vi "radar.vi"(0 "Radar configuration":string="{\n\t\"type\": \"Radar\",\n\t\"gpu_number\": 0,\n\t\"listen_port\": 8302,\n\t\"send_radar_cube\": false,\n\t\"paint_targets\": false,\n\t\"run_tracker\": true,\n\t\"tracker\": {\n\t\t\"cluster_threshold\": 1.0,\n\t\t\"filter_size\": 8,\n\t\t\"kalman_alpha\": 10.0,\n\t\t\"kinematic_iir_alpha\": 0.05000000074505806,\n\t\t\"min_cluster_distance\": 25.0,\n\t\t\"min_detections_per_cluster\": 2,\n\t\t\"missed_detections_threshold\": 5,\n\t\t\"vel_coeff\": 0.699999988079071,\n\t\t\"write_debug_json\": \"\",\n\t\t\"x_dir_coeff\": 9.0,\n\t\t\"y_dir_coeff\": 4.199999809265137\n\t},\n\t\"rois\": [{\n\t\t\"max_angle\": 10.0,\n\t\t\"max_range\": 20.0,\n\t\t\"min_angle\": 0.0,\n\t\t\"min_range\": 1.0,\n\t\t\"roi_name\": \"test_left_roi\"\n\t}, {\n\t\t\"max_angle\": 0.0,\n\t\t\"max_range\": 20.0,\n\t\t\"min_angle\": -10.0,\n\t\t\"min_range\": 1.0,\n\t\t\"roi_name\": \"test_right_roi\"\n\t}],\n\t\"target_paint_lifetime\": 0.5,\n\t\"nearest_target_label_radius\": 100.0,\n\t\"location\": {\n\t\t\"x\": 245.0,\n\t\t\"y\": 0.0,\n\t\t\"z\": 40.0\n\t},\n\t\"rotation\": {\n\t\t\"pitch\": 0.0,\n\t\t\"yaw\": 0.0,\n\t\t\"roll\": 0.0\n\t},\n\t\"num_samples_per_sweep\": 345,\n\t\"fs\": 50000000,\n\t\"fc\": 77000000000.0,\n\t\"num_sweeps\": 16,\n\t\"sweep_time\": 0.0000069,\n\t\"bandwidth\": 250000000,\n\t\"max_radar_returns\": 500,\n\t\"elements\": 8,\n\t\"transmitter\": {\n\t\t\"peak_power\": 5.0,\n\t\t\"aperture\": 0.000859,\n\t\t\"gain\": 13.50\n\t},\n\t\"receiver\": {\n\t\t\"aperture\": 0.000798,\n\t\t\"nf\": 10.0,\n\t\t\"noise_temp\": 290.0,\n\t\t\"nb\": 74000000.0,\n\t\t\"gain\": 10.0\n\t},\n\t\"sbr\": {\n\t\t\"long_range_scan_distance\": 100.0,\n\t\t\"short_range_scan_distance\": 30.0,\n\t\t\"long_range_fov\": 30.0,\n\t\t\"short_range_fov\": 60.0,\n\t\t\"elevation_fov\": 10.0,\n\t\t\"ray_division_y\": 10.0,\n\t\t\"ray_division_z\": 10.0,\n\t\t\"debug_frustum\": false,\n\t\t\"debug_scan\": false,\n\t\t\"debug_rescan\": false\n\t}\n}", 3 "error in":errorcluster) -> (4 "Radar configuration":string="[\n    {\n  \"type\": \"Radar\",\n  \"packet_size\": 64000,\n   \"gpu_number\":0,\n  \"listen_port\": 8301,\n  \"synchronized_display\": true,\n  \"paint_targets\": false,\n  \"target_paint_lifetime\": 0.5,\n  \"location\": {\n    \"x\": 250.0,\n    \"y\": 0.0,\n    \"z\": 50.0\n  },\n  \"rotation\": {\n    \"pitch\": 0.0,\n    \"yaw\": 0.0,\n    \"roll\": 0.0\n  },\n  \"num_samples_per_sweep\":345,\n  \"fs\": 50000000,\n  \"fc\": 77000000000.0,\n  \"num_sweeps\": 32,\n  \"sweep_time\" : 0.0000069,\n  \"bandwidth\" : 172500000,\n  \"max_targets\": 250,\n  \"elements\": 8,\n  \"transmitter\": {\n    \"peak_power\": 5.0,\n    \"aperture\": 0.000859,\n    \"gain\": 13.50\n  },\n  \"receiver\": {\n    \"aperture\": 0.000798,\n    \"nf\": 10.0,\n    \"noise_temp\": 290.0,\n    \"nb\": 74000000.0,\n    \"gain\": 10.0\n  },\n  \"sbr\": {\n    \"long_range_scan_distance\": 150.0,\n    \"short_range_scan_distance\": 60.0,\n    \"long_range_fov\": 20.0,\n    \"short_range_fov\": 60.0,\n    \"elevation_fov\": 10.0,\n    \"rescan_density\": 20.0,\n    \"debug_frustum\": false,\n    \"debug_scan\": false,\n    \"debug_rescan\": false\n  }\n}\n]", 5 "Radar Sample":T2, 6 "Radar Data Cube":string, 7 "Target list":string, 8 "error out":errorcluster)   [LabVIEW 2019]
doc: "Configure and reads the data stream for the Radar sensor.\ns"
uses:
  tools/simx_common.vi
  controls/radarSample.ctl
  controls/RadarTrack.ctl
  controls/Header.ctl
panel:
  out "Header":T1
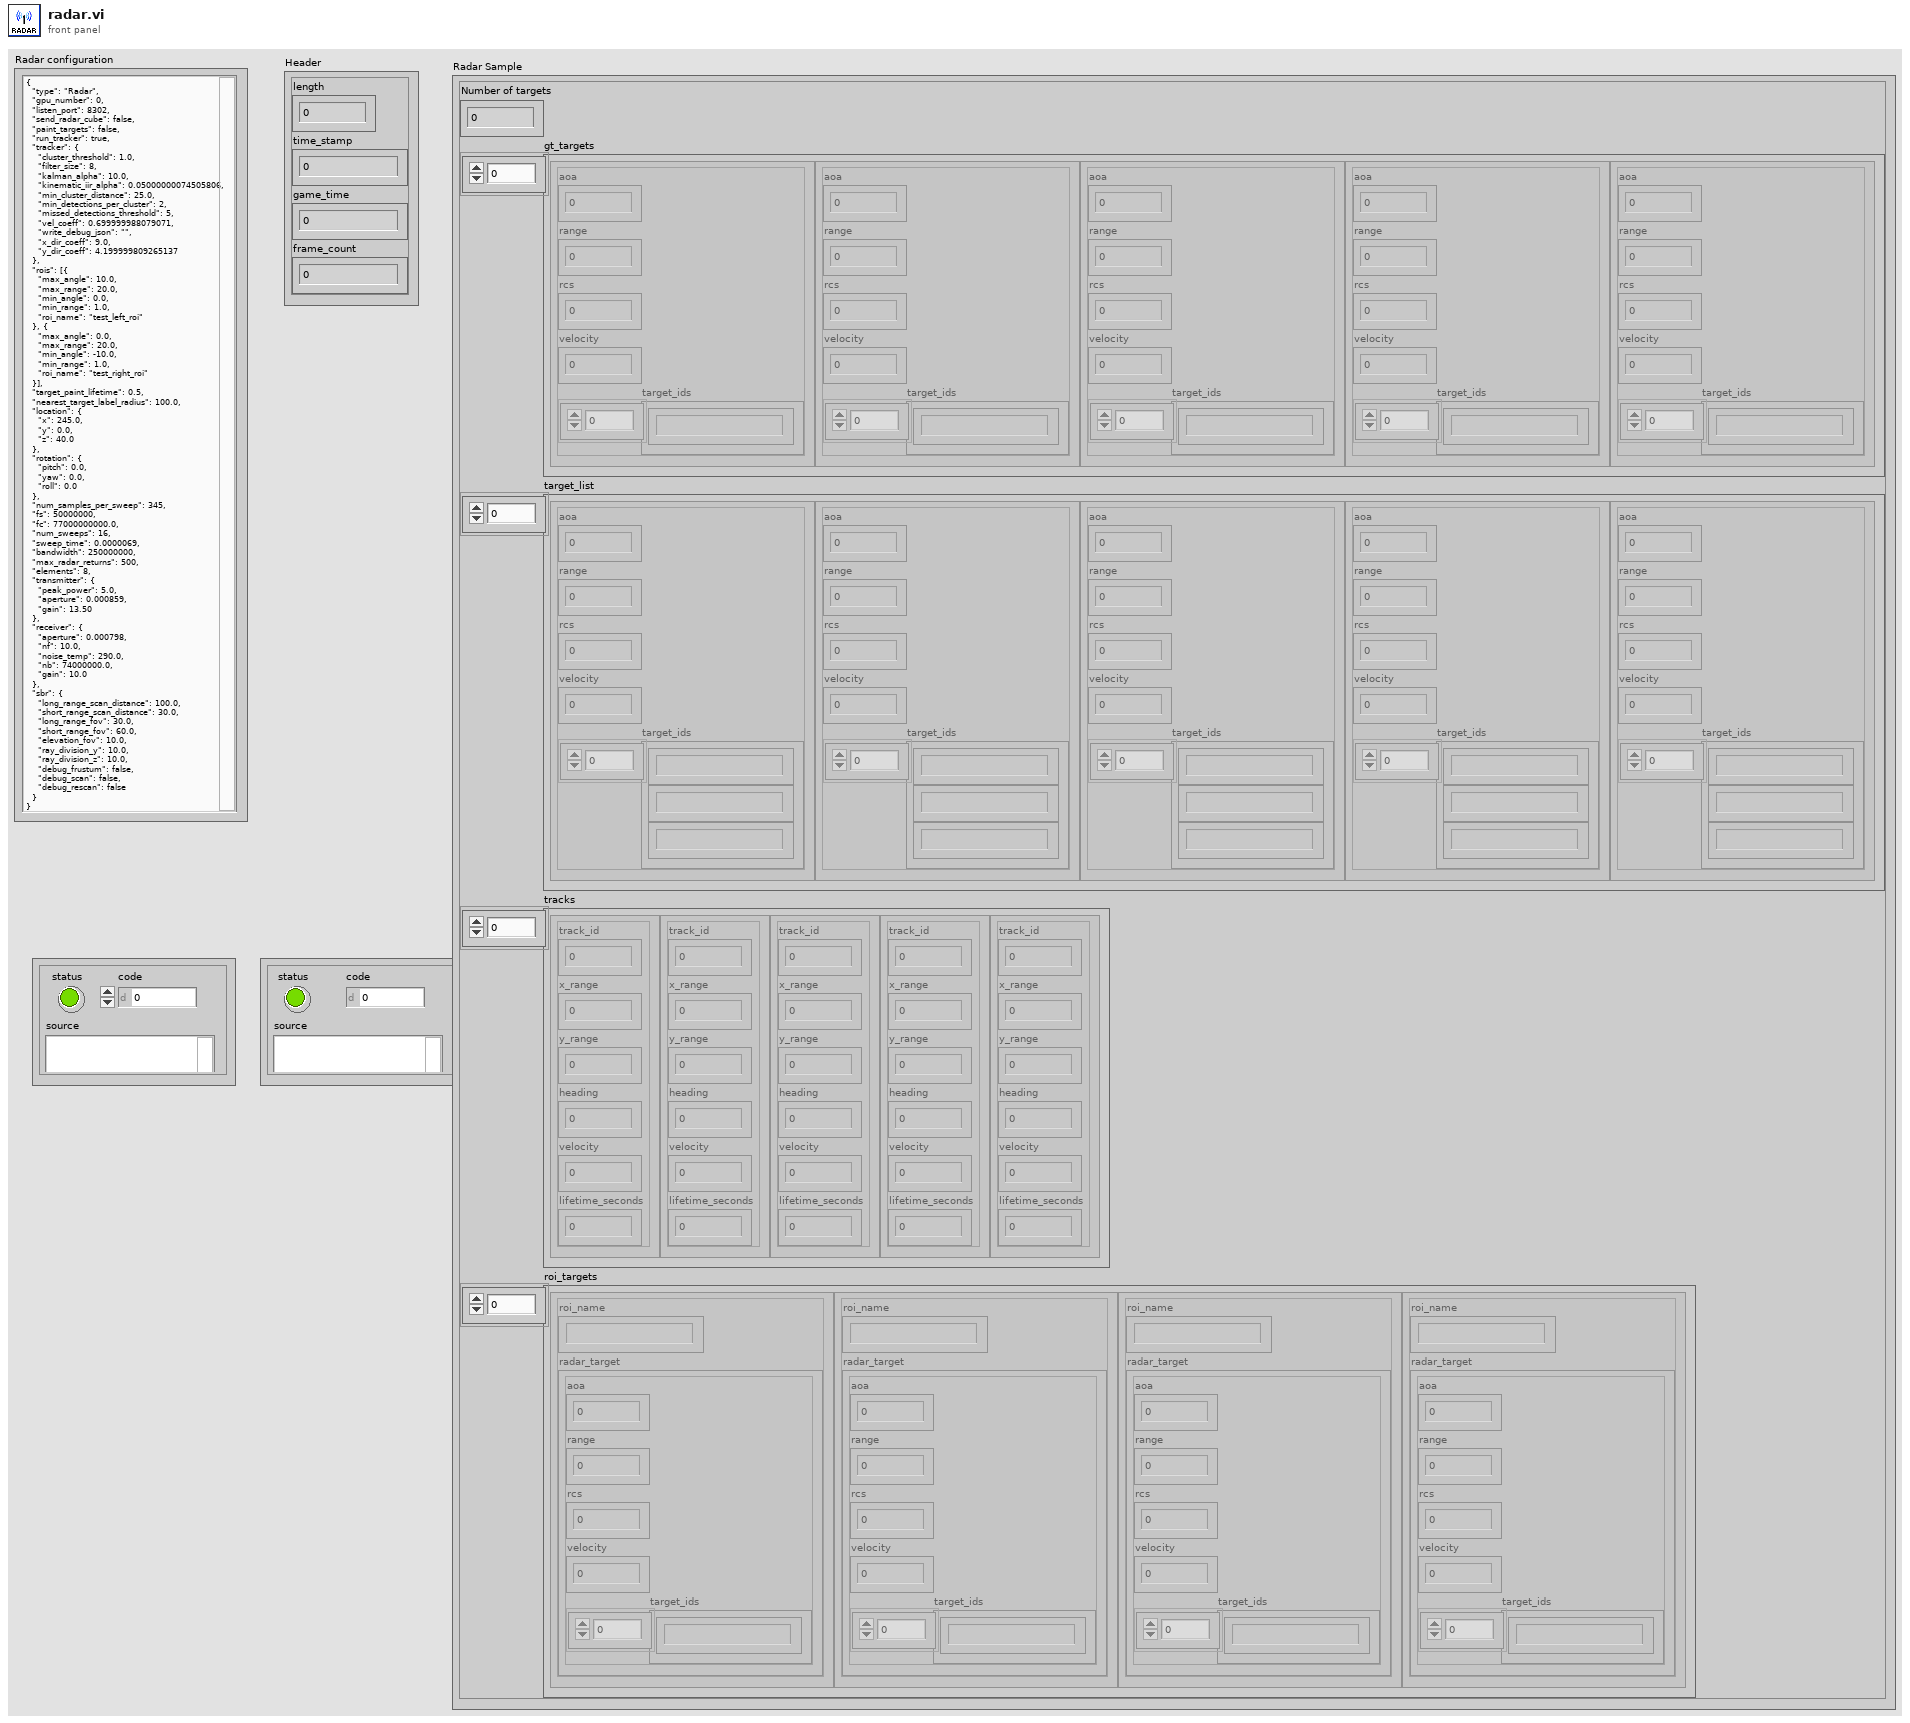
[diagram p1: front panel]
types:
  T1 = typedef "Header.ctl" = cluster{"length":u32, "time_stamp":u32, "game_time":sgl, "frame_count":u32}
  T2 = typedef "radarSample.ctl" = cluster{"Number of targets":i32, "gt_targets":cluster{"aoa":sgl, "range":sgl, "rcs":sgl, "velocity":sgl, "target_ids":string[]}[], "target_list":cluster{"aoa":sgl, "range":sgl, "rcs":sgl, "velocity":sgl, "target_ids":string[]}[], "tracks":T3[], "roi_targets":cluster{"roi_name":string, "radar_target":cluster{"aoa":sgl, "range":sgl, "rcs":sgl, "velocity":sgl, "target_ids":string[]}}[]}
  T3 = typedef "RadarTrack.ctl" = cluster{"track_id":u64, "x_range":sgl, "y_range":sgl, "heading":sgl, "velocity":sgl, "lifetime_seconds":sgl}
  T4 = typedef "simx_connection.ctl" = cluster{"Config":T5, "Connections":T8, "Map":cluster{"lanes":cluster{"x":dbl[], "y":dbl[], "z":dbl[]}, "StartPosition":cluster{"start_points":T9, "StartRotation":dbl[], "StartLocation":dbl[]}, "Draw Map Size":T10, "DrawArea":cluster{"min_Y":dbl, "min_X":dbl, "Scale X":dbl, "Scale Y":dbl}, "Map":picture, "Map Geojson":string}}
  T5 = typedef "config.ctl" = cluster{"Trajectory":T6, "Weather":T7}
  T6 = typedef "trajectory.ctl" = cluster{"Number of frames":i32, "Frame number":i32, "Trajectory":string}
  T7 = typedef "weather.ctl" = cluster{"id":string}
  T8 = typedef "connections.ctl" = cluster{"Simulator Connection":refnum<k5>, "server_ip":string, "Port":i32, "Sensor connections":refnum<k5>[]}
  T9 = typedef "start_points.ctl" = cluster{"locations":dbl[][], "rotations":dbl[][], "type":string[]}
  T10 = typedef "LVBoundsTypeDef.ctl" = cluster{"Width":u32, "Height":u32}
  T11 = typedef "sensor_sample.ctl" = cluster{"Header":T1, "data out":string}
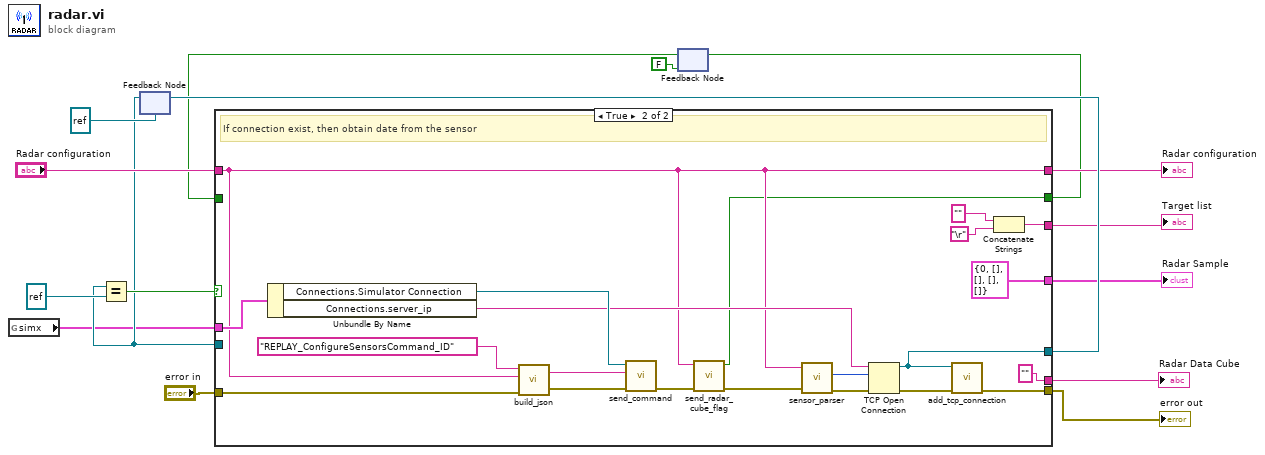
[diagram p0: block diagram]
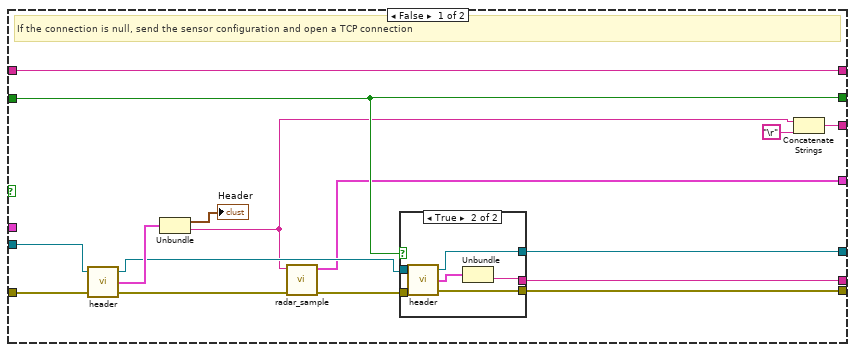
[diagram p2: hidden frame]
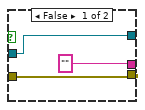
[diagram p3: hidden frame]
diagram:
  n1 = global read "simx_common.vi" "simx"() -> (w3:T4)
  n2 = feedback #1(refnum<k5> refnum ("radar_connection")) -> (w10:refnum<k5>)
  n3 = Equal?(x=w10, y=refnum<k5> refnum ("null connection")) -> (x = y?=w12:bool)
  n4 = feedback #2(FALSE ("send_radar_cube")) -> (w6:bool)
  n5 = case shown="True" w12 {
    tunnel: [w28 w58] -> w16
    tunnel: "Radar configuration" -> [w26 w48]
    tunnel: [w27 w57] -> w13
    tunnel: w10 -> [w30 _]
    tunnel: "error in" -> [w29 w53]
    tunnel: [w26 w48] -> w8
    tunnel: [w25 w47] -> w7
    tunnel: w6 -> [w25 _]
    tunnel: [w21 T2 {"Number of targets"=0, "gt_targets"=[], "target_list"=[], "tracks"=[], "roi_targets"=[]} ("Radar")] -> w4
    tunnel: w3 -> [_ w56]
    tunnel: [w17 "" ("data out")] -> w2
    tunnel: [w18 w43] -> w1
    frame False {
      # "If the connection is null, send the sensor configuration and open a TCP connection"
      n6 = call "header.vi"("error in"=w29, "TCP Network Connection in"=w30) -> ("error out"=w23:errorcluster, "Sensor sample"=w32:T11, "TCP Network Connection out"=w31:refnum<k5>)  [unwired: 1 in]
      n7 = Unbundle(w32) -> ("Header"=→"Header":T1, "data out"=w24:string)
      n8 = call "radar_sample.vi"("error in"=w23, "Raw data"=w24) -> ("error out"=w22:errorcluster, "Radar Sample"=w21:T2)  [unwired: 4 in]
      n9 = case shown="True" w25 {
        tunnel: w22 -> [w34 w41]
        tunnel: w31 -> [w35 w40]
        tunnel: [w34 w39] -> w28
        tunnel: [w35 w38] -> w27
        tunnel: ["" ("data out") w36] -> w17
        frame False {
        }
        frame True {
          n10 = call "header.vi"("error in"=w41, "TCP Network Connection in"=w40) -> ("error out"=w39:errorcluster, "Sensor sample"=w37:T11, "TCP Network Connection out"=w38:refnum<k5>)  [unwired: 1 in]
          n11 = Unbundle(w37) -> ("data out"=w36:string)  [unwired: 1 out]
        }
      }
      n12 = Concatenate Strings(w24, "\r") -> (w18:string)
    }
    frame True {
      # "If connection exist, then obtain date from the sensor"
      n13 = Unbundle By Name(w56) -> ("Connections.Simulator Connection"=w55:refnum<k5>, "Connections.server_ip"=w54:string)
      n14 = call "build_json.vi"("error in"=w53, "Message"=w48, "Command_ID"="REPLAY_ConfigureSensorsCommand_ID") -> ("error out"=w60:errorcluster, "JSON Out"=w61:string)  [unwired: 1 in]
      n15 = call "send_command.vi"("error in"=w60, "JSON Command"=w61, "TCP Network Connection in"=w55) -> ("error out"=w52:errorcluster)  [unwired: 1 in, 3 out]
      n16 = call "send_radar_cube_flag.vi"("error in"=w52, "Radar configuration"=w48) -> ("error out"=w51:errorcluster, "send_radar_cube"=w47:bool)  [unwired: 4 in]
      n17 = call "sensor_parser.vi"("Sensor configuration"=w48, "error in"=w51) -> ("Port out"=w49:u16, "error out"=w50:errorcluster)  [unwired: 1 in, 2 out]
      n18 = TCP Open Connection(address=w54, remote port or service name=w49, error in (no error)=w50) -> (connection ID=w57:refnum<k5>, error out=w59:errorcluster)  [unwired: 2 in]
      n19 = call "add_tcp_connection.vi"("error in"=w59, "Sensor connection"=w57) -> ("error out"=w58:errorcluster)  [unwired: 5 in]
      n20 = Concatenate Strings("" ("data out"), "\r") -> (w43:string)
    }
  }
  "error out" <- w16
  "Radar Data Cube" <- w2
  "Radar configuration" <- w8
  "Target list" <- w1
  "Radar Sample" <- w4
  n21 = feedback-in #1(w13) -> ()
  n22 = feedback-in #2(w7) -> ()
